vi "Autosize Listbox Columns (Uniform Text).vi"(4 "error in (no error)":errorcluster, 6 "Resize Table?":bool, 7 "Table Ref":refnum<vi>) -> (0 "error out":errorcluster)   [LabVIEW 2016]
doc: "This VI resizes each column of the table specified by Table Ref based on the widest entry of the column. Additionally, if Resize Table? is TRUE, the VI will set the table width based on the number of populated columns."
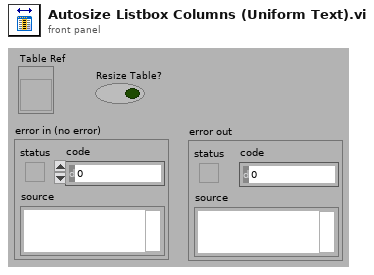
[diagram p1: front panel]
types:
  T1 = enum16{"User-specified Font", "Application Font", "System Font", "Dialog Font"}
  T2 = cluster{"Font Name:":string, "Size":i16, "Strikeout?":bool, "Italic?":bool, "Underline?":bool, "Outline?":bool, "Shadow?":bool, "Bold?":bool}
  T3 = cluster{"left":i16, "top":i16, "right":i16, "bottom":i16}
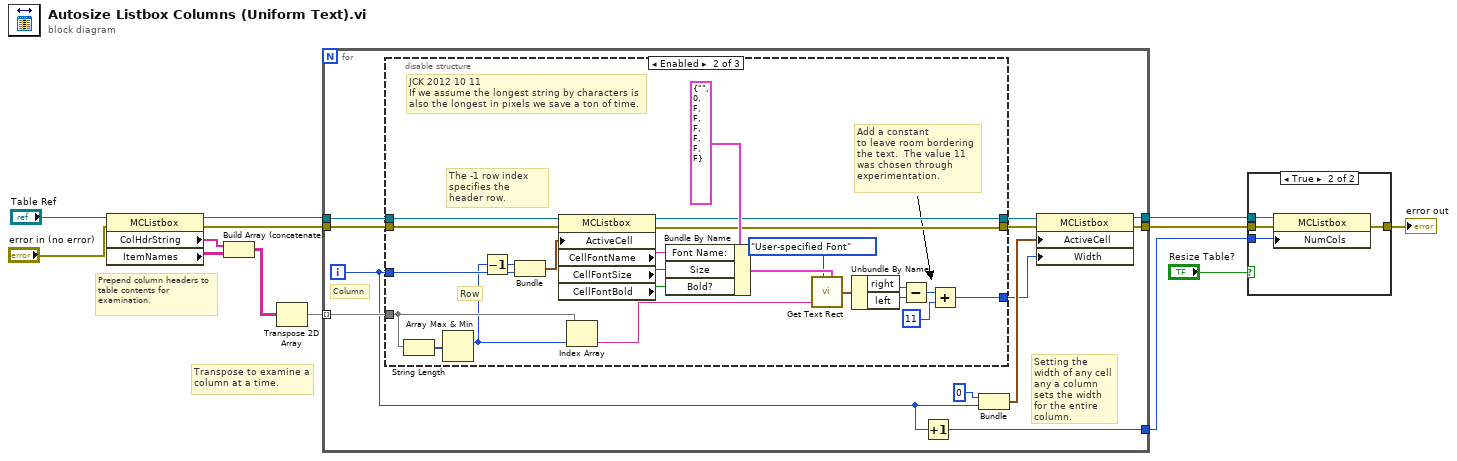
[diagram p0: block diagram]
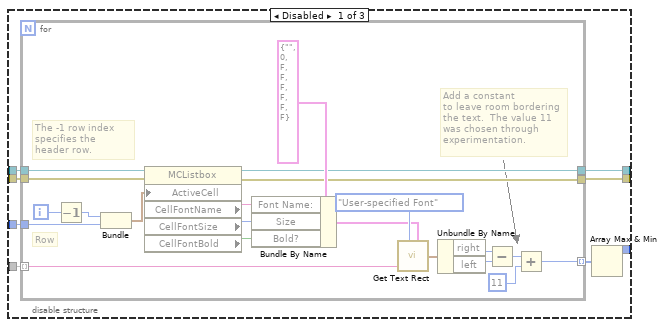
[diagram p3: hidden frame]
diagram:
  # "Transpose to examine a column at a time."
  # "Prepend column headers to table contents for examination."
  n1 = property class="MCListbox"(reference="Table Ref", error in="error in (no error)") -> (reference out=w13:refnum<vi>, error out=w9:errorcluster, "ColHdrString"=w12:string[], "ItemNames"=w8:string[][])
  n2 = Build Array (concatenate)(w12, w8) -> (w11:string[][])
  n3 = Transpose 2D Array(2D array=w11) -> (transposed array=w10:string[][])
  n4 = for {
    tunnel: w10 -> [w25] mode=indexing
    tunnel: w13 -> [w24]
    tunnel: w9 -> [w23]
    tunnel: [w17] -> w3
    tunnel: [w16] -> w4
    tunnel: [w14] -> w2
    i -> [w15]
    # "Setting the width of any cell any a column sets the width for the entire column."
    # "Column"
    n5 = disable-structure shown="Enabled" {
      disable-tunnel: w25 -> [w33 w62 _]
      disable-tunnel: w24 -> [w32 w59 _]
      disable-tunnel: w23 -> [w30 w58 _]
      disable-tunnel: [w29 w57 _] -> w22
      disable-tunnel: [w28 w56 _] -> w21
      disable-tunnel: [w27 w55 _] -> w18
      disable-tunnel: w15 -> [w26 w63 _]
      frame Disabled {
        n6 = for {
          tunnel: w33 -> [w46] mode=indexing
          tunnel: w32 -> [w54]
          tunnel: w26 -> [w53]
          tunnel: [w35] -> w31 mode=indexing
          tunnel: w30 -> [w40]
          tunnel: [w39] -> w28
          tunnel: [w38] -> w29
          i -> [w42]
          # "The -1 row index specifies the header row."
          # "Add a constant\nto leave room bordering the text.  The value 11 was chosen through experimentation."
          # "Row"
          n7 = Decrement(x=w42) -> (x-1=w41:i32)
          n8 = Bundle(w41, w53) -> (w52:cluster{i32, i32})  [unwired: 1 in]
          n9 = property class="MCListbox"(reference=w54, error in=w40, "ActiveCell"=w52) -> (reference out=w38:refnum<vi>, error out=w39:errorcluster, "CellFontName"=w50:string, "CellFontSize"=w36:u32, "CellFontBold"=w49:bool)
          n10 = Bundle By Name(cluster=T2 {"Font Name:"="", "Size"=0, "Strikeout?"=FALSE, "Italic?"=FALSE, "Underline?"=FALSE, "Outline?"=FALSE, "Shadow?"=FALSE, "Bold?"=FALSE} ("[user-specified font]"), "Font Name:"=w50, "Size"=w36, "Bold?"=w49) -> (w47:T2)
          n11 = call <vilib>:"Get Text Rect.vi"("desired font(Application)"=T1."User-specified Font", "text"=w46, "[user-specified font]"=w47) -> ("rect"=w45:T3)  [unwired: 6 in]
          n12 = Unbundle By Name(w45) -> ("right"=w44:i16, "left"=w43:i16)
          n13 = Subtract(x=w44, y=w43) -> (x-y=w37:i16)
          n14 = Add(x=w37, y=i16 11) -> (x+y=w35:i16)
        }
        n15 = Array Max & Min(array=w31) -> (max value=w27:i16)  [unwired: 3 out]
      }
      frame Enabled {
        # "JCK 2012 10 11\nIf we assume the longest string by characters is also the longest in pixels we save a ton of time."
        # "The -1 row index specifies the header row."
        # "Add a constant\nto leave room bordering the text.  The value 11 was chosen through experimentation."
        # "Row"
        n16 = String Length(string=w62) -> (length=w77:i32[])
        n17 = Array Max & Min(array=w77) -> (max index (indices)=w61:i32)  [unwired: 3 out]
        n18 = Decrement(x=w61) -> (x-1=w73:i32)
        n19 = Bundle(w73, w63) -> (w64:cluster{i32, i32})  [unwired: 1 in]
        n20 = property class="MCListbox"(reference=w59, error in=w58, "ActiveCell"=w64) -> (reference out=w57:refnum<vi>, error out=w56:errorcluster, "CellFontName"=w66:string, "CellFontSize"=w75:u32, "CellFontBold"=w67:bool)
        n21 = Index Array(array=w62, index=w61) -> (element=w60:string)
        n22 = Bundle By Name(cluster=T2 {"Font Name:"="", "Size"=0, "Strikeout?"=FALSE, "Italic?"=FALSE, "Underline?"=FALSE, "Outline?"=FALSE, "Shadow?"=FALSE, "Bold?"=FALSE} ("[user-specified font]"), "Font Name:"=w66, "Size"=w75, "Bold?"=w67) -> (w69:T2)
        n23 = call <vilib>:"Get Text Rect.vi"("desired font(Application)"=T1."User-specified Font", "text"=w60, "[user-specified font]"=w69) -> ("rect"=w70:T3)  [unwired: 6 in]
        n24 = Unbundle By Name(w70) -> ("right"=w71:i16, "left"=w72:i16)
        n25 = Subtract(x=w71, y=w72) -> (x-y=w74:i16)
        n26 = Add(x=w74, y=i16 11) -> (x+y=w55:i16)
      }
      frame Disabled {
      }
    }
    n27 = Increment(x=w15) -> (x+1=w14:i32)
    n28 = Bundle(0, w15) -> (w19:cluster{i32, i32})  [unwired: 1 in]
    n29 = property class="MCListbox"(reference=w22, error in=w21, "ActiveCell"=w19, "Width"=w18) -> (reference out=w16:refnum<vi>, error out=w17:errorcluster)
  }
  n30 = case shown="True" "Resize Table?" {
    tunnel: w4 -> [_ w82]
    tunnel: w3 -> [w78 w81]
    tunnel: w2 -> [_ w80]
    tunnel: [w78 w79] -> w1
    frame False {
    }
    frame True {
      n31 = property class="MCListbox"(reference=w82, error in=w81, "NumCols"=w80) -> (error out=w79:errorcluster)  [unwired: 1 out]
    }
  }
  "error out" <- w1
